vi "ERR HANDLER - CMD Q.vi"() -> (3 "Err Handler Q":refnum<queue>)   [LabVIEW 2013]
uses:
  Error Queue Message.ctl
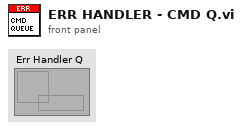
[diagram p1: front panel]
types:
  T1 = typedef "Error Queue Message.ctl" = cluster{"Command":enum16{"HANDLE ERROR", "EXIT"}, "Data":variant}
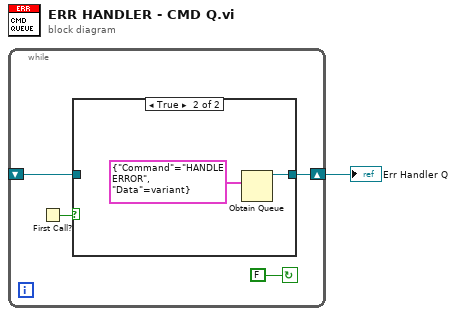
[diagram p0: block diagram]
diagram:
  n1 = while {
    shift-right: [w3] -> w1
    shift-left: _ -> [w2]
    stop <- FALSE continue-if-true
    n2 = First Call?() -> (First Call?: T/F=w4:bool)
    n3 = case shown="True" w4 {
      tunnel: [w6 w7] -> w3
      tunnel: w2 -> [w6 _]
      frame False {
      }
      frame True {
        n4 = Obtain Queue(element data type=T1 {"Command"=enum."HANDLE ERROR", "Data"=variant} ("Error Handler Mesg")) -> (queue out=w7:refnum<queue>)  [unwired: 4 in, 2 out]
      }
    }
  }
  "Err Handler Q" <- w1
